vi "Msg Output Terminals.vi"(10 "Msg Output Terminals":i32[](array[numeric])) -> (1 "Read Msg Output Terminals":i32[](array[numeric]), 2 "Init Msg Output Terminals":i32[](array[numeric]))   [LabVIEW 2025, in "_Rescript.lvlib" / "Msg.lvlib"]
uses:
  Msg.lvlib
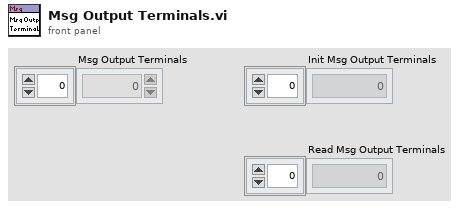
[diagram p1: front panel]
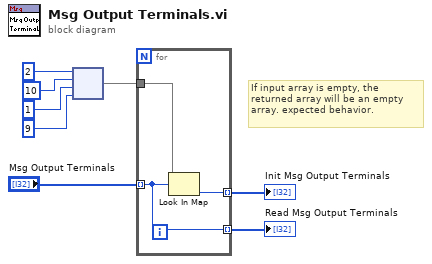
[diagram p0: block diagram]
diagram:
  # "If input array is empty, the returned array will be an empty array. expected behavior."
  n1 = node(2 ("Numeric"), 10 ("Numeric"), 1 ("Numeric"), 9 ("Numeric")) -> (w2:map{i32, i32})
  n2 = for {
    tunnel: [w10] -> w8 mode=indexing
    tunnel: "Msg Output Terminals" -> [w9] mode=indexing
    tunnel: w2 -> [w11]
    tunnel: [w9] -> w1 mode=indexing
    n3 = Look In Map(map=w11, key=w9) -> (value=w10:i32)  [unwired: 1 in, 1 out]
  }
  "Init Msg Output Terminals" <- w8
  "Read Msg Output Terminals" <- w1
